vi "OutputChannels.vi"(1 "Get/Set":bool, 2 "Output Channels (input)":tag) -> (0 "Output Channels (output)":tag)   [LabVIEW 2009]
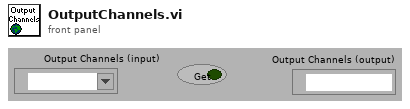
[diagram p1: front panel]
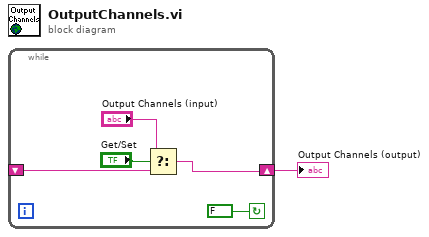
[diagram p0: block diagram]
diagram:
  n1 = while {
    shift-right: [w4] -> w1
    shift-left: _ -> [w5]
    stop <- FALSE continue-if-true
    n2 = Select(t="Output Channels (input)", s="Get/Set", f=w5) -> (s? t:f=w4:tag)
  }
  "Output Channels (output)" <- w1
